vi "CLD 9 Step Sequencer Express Timer Front Panel.vi"() -> ()   [LabVIEW 2018]
doc: "CLD 9 Exercise"
uses:
  CLD 9 Timer Enum.ctl
panel:
  out "Current Step Time":dbl
  out "Elapsed Time (s)":string
  out "Step 3":bool
  out "Step 2":bool
  out "Step 1":bool
  out "Time Has Elapsed":bool
  in  "Auto Reset":bool=TRUE
  in  "Reset Button":bool
  in  "Stop VI":bool
  out "error out":errorcluster
  in  "error in (no error)":errorcluster
  in  "Time Target (s)":dbl
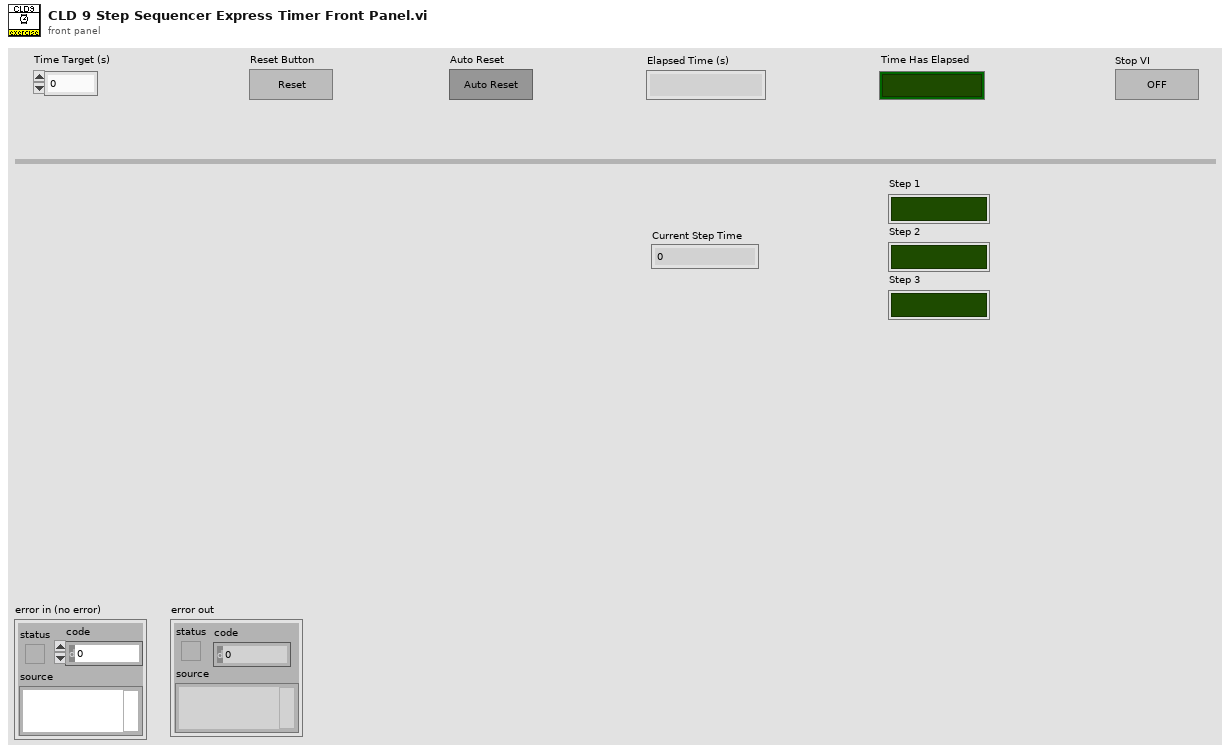
[diagram p1: front panel]
types:
  T1 = typedef "CLD 9 Timer Enum.ctl" = enum16{"Run Step One", "Run Step Two", "Run Step Three"}
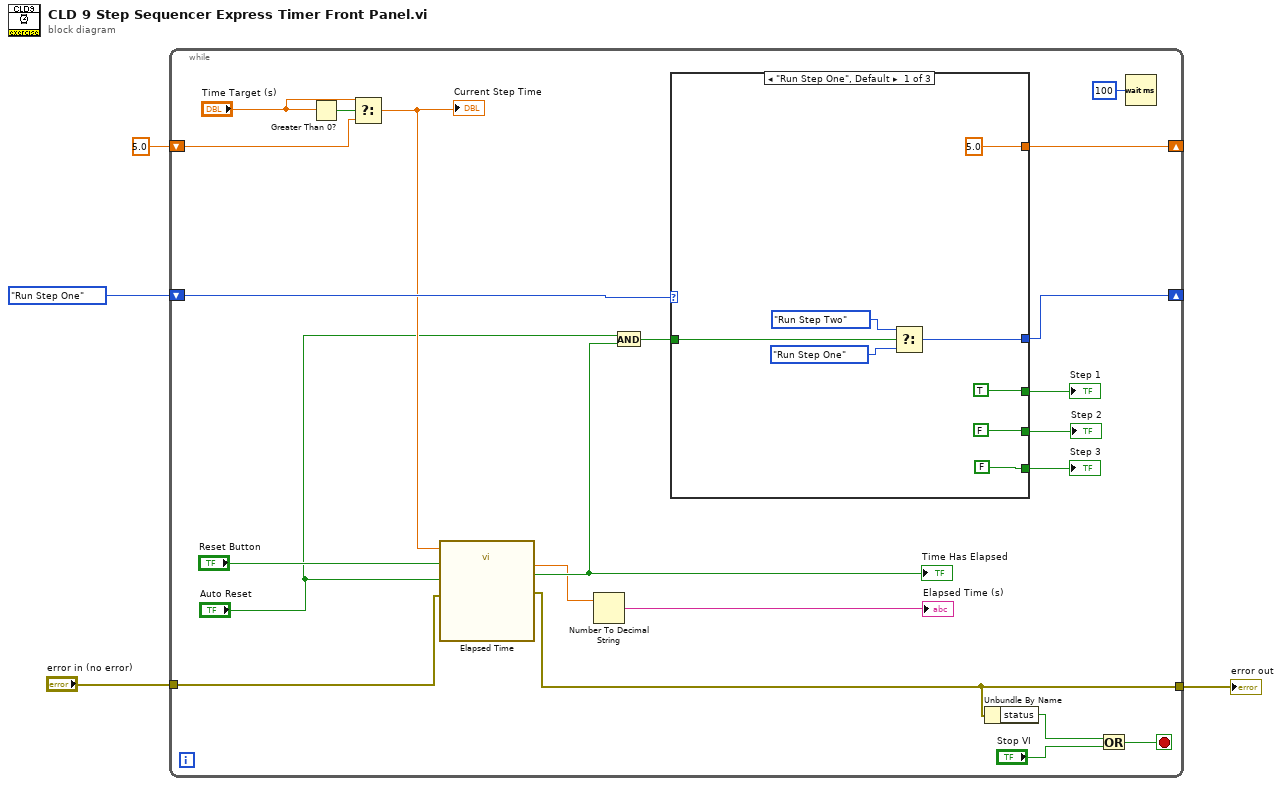
[diagram p0: block diagram]
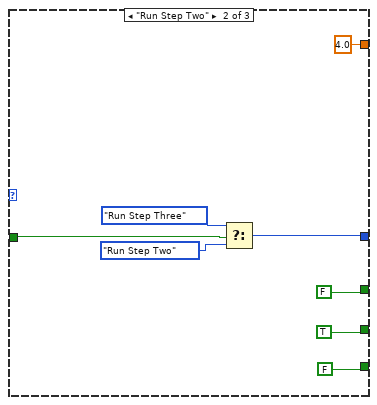
[diagram p2: hidden frame]
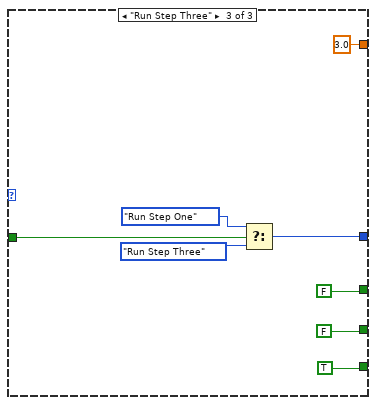
[diagram p3: hidden frame]
diagram:
  n1 = while {
    shift-right: [w21] -> _
    shift-left: CLD_9_Timer_Enum."Run Step One" ("CLD 9 Timer Enum") -> [w26]
    shift-right: [w20] -> _
    shift-left: 5.0 ("f") -> [w23]
    tunnel: "error in (no error)" -> [w19]
    tunnel: [w18] -> w1
    stop <- w15 stop-if-true
    n2 = Greater Than 0?(x="Time Target (s)") -> (x > 0?=w25:bool)
    n3 = Select(t="Time Target (s)", s=w25, f=w23) -> (s? t:f=w22:dbl)
    "Current Step Time" <- w22
    n4 = call "Elapsed Time"("Time Target (s)"=w22, "Reset"="Reset Button", "Auto Reset"="Auto Reset", "error in (no error)"=w19) -> ("Elapsed Time (s)"=w6:dbl, "Time has Elapsed"=w9:bool, "error out"=w18:errorcluster)  [unwired: 8 in, 5 out]
    "Time Has Elapsed" <- w9
    n5 = Number To Decimal String(number=w6) -> (decimal integer string=→"Elapsed Time (s)":string)  [unwired: 1 in]
    n6 = And(x="Auto Reset", y=w9) -> (x .and. y?=w10:bool)
    n7 = case shown="\"Run Step One\", Default" w26 {
      tunnel: w10 -> [w34 w37 w45]
      tunnel: [w32 w36 w44] -> w21
      tunnel: [5.0 ("f") 4.0 ("f") 3.0 ("f")] -> w20
      tunnel: [TRUE FALSE FALSE] -> w14
      tunnel: [FALSE TRUE FALSE] -> w13
      tunnel: [FALSE FALSE TRUE] -> w12
      frame "Run Step One", Default {
        n8 = Select(t=CLD_9_Timer_Enum."Run Step Two" ("CLD 9 Timer Enum"), s=w34, f=CLD_9_Timer_Enum."Run Step One" ("CLD 9 Timer Enum")) -> (s? t:f=w32:T1)
      }
      frame "Run Step Two" {
        n9 = Select(t=CLD_9_Timer_Enum."Run Step Three" ("CLD 9 Timer Enum"), s=w37, f=CLD_9_Timer_Enum."Run Step Two" ("CLD 9 Timer Enum")) -> (s? t:f=w36:T1)
      }
      frame "Run Step Three" {
        n10 = Select(t=CLD_9_Timer_Enum."Run Step One" ("CLD 9 Timer Enum"), s=w45, f=CLD_9_Timer_Enum."Run Step Three" ("CLD 9 Timer Enum")) -> (s? t:f=w44:T1)
      }
    }
    "Step 1" <- w14
    "Step 2" <- w13
    "Step 3" <- w12
    n11 = Unbundle By Name(w18) -> ("status"=w17:bool)
    n12 = Or(x=w17, y="Stop VI") -> (x .or. y?=w15:bool)
    n13 = Wait (ms)(milliseconds to wait=u32 100) -> ()  [unwired: 1 out]
  }
  "error out" <- w1
